vi "00 Main Simulated Signal (x64-2018).vi"() -> ()   [LabVIEW 2017]
panel:
  out "Error out (DAQ Loop)":errorcluster
  out "DAQ Loop Iterations":i32
  out "Raw DAQ Output":dynamicdata(graph)=[{"t0"=timestamp(3367839419.335167 s since 1904-01-01), "dt"=0.00016666666666666663, "Y"=array[240 elements], "attributes"=variant("NI_ChannelName"=variant(string "Voltage_0"), "NI_UnitDescription"=variant(string "Volts"))}, {"t0"=timestamp(3367839419.3351874 s since 1904-01-01), "dt"=0.00016666666666666663, "Y"=array[240 elements], "attributes"=variant("NI_ChannelName"=variant(string "Voltage_1"), "NI_UnitDescription"=variant(string "Volts"))}, {"t0"=timestamp(3367839419.3352084 s since 1904-01-01), "dt"=0.00016666666666666663, "Y"=array[240 elements], "attributes"=variant("NI_ChannelName"=variant(string "Voltage_2"), "NI_UnitDescription"=variant(string "Volts"))}]
  in  "All Stop!":bool
  out "Frequency 2":dynamicdata(graph)=[{"t0"=timestamp(3424329819.6880417 s since 1904-01-01), "dt"=0.00016666666666666663, "Y"=[50.00644377121546], "attributes"=variant("NI_ChannelName"=variant(string "Detected Frequency"))}, {"t0"=timestamp(3424329819.6880627 s since 1904-01-01), "dt"=0.00016666666666666663, "Y"=[49.993846178541475], "attributes"=variant("NI_ChannelName"=variant(string "Detected Frequency"))}, {"t0"=timestamp(3424329819.6880836 s since 1904-01-01), "dt"=0.00016666666666666663, "Y"=[49.994041382621866], "attributes"=variant("NI_ChannelName"=variant(string "Detected Frequency"))}] caption="Frequency"
  out "Phase 2":dynamicdata(graph)=[{"t0"=timestamp(3424329819.6880417 s since 1904-01-01), "dt"=0.00016666666666666663, "Y"=[-19.090260250465658], "attributes"=variant("NI_ChannelName"=variant(string "Detected Phase"))}, {"t0"=timestamp(3424329819.6880627 s since 1904-01-01), "dt"=0.00016666666666666663, "Y"=[-138.45601955575555], "attributes"=variant("NI_ChannelName"=variant(string "Detected Phase"))}, {"t0"=timestamp(3424329819.6880836 s since 1904-01-01), "dt"=0.00016666666666666663, "Y"=[102.37498697247455], "attributes"=variant("NI_ChannelName"=variant(string "Detected Phase"))}] caption="Frequency"
  out "Frequency":dbl format="%.2f"
  out "Amplitude":dbl format="%.2f"
  out "Phase":dbl format="%.2f"
  out "Acquisition Time":timestamp
  out "Voltage Waveform":dynamicdata(graph)=[{"t0"=timestamp(3424329819.638042 s since 1904-01-01), "dt"=0.00016666666666666663, "Y"=array[300 elements]}, {"t0"=timestamp(3424329819.6380625 s since 1904-01-01), "dt"=0.00016666666666666663, "Y"=array[300 elements]}, {"t0"=timestamp(3424329819.6380835 s since 1904-01-01), "dt"=0.00016666666666666663, "Y"=array[300 elements]}]
  out "IP":string
  out "Port":i32
  out "Transmitted Data":string
  out "Stop":bool
  out "Elements in Acquisition Buffer":i32
  # "V1.2 - PFI0 (Three Phase)"
  # "50.5"
  # "Rate"
  # "49.5"
  # "The code and design of this VI are licensed \nunder the terms of the New BSD License.\nPlease see the VI documentation or License.txt\nfor more details.\n\nCopyright (c) 2012, David Laverty\nwww.OpenPMU.org"
  # "180"
  # "-180"
  # "Configuration Information:\n\nThe ID and IP address to which the OpenPMU sends data is configured by 'C:\\PMUconfig.ini'.  If this doesn't exist, create it.\n\nCopy and paste the blue text below without the dashed lines into PMUconfig.ini.\n\n[Telecoms]\nID=PMU123\nIP=192.168.1.100\nPort=40001\n\nIP and Port may be any values within normal IPv4 range.  ID should be six alpha-numeric characters."
  # "Debug Stuff ( you're not supposed to find this :P )"
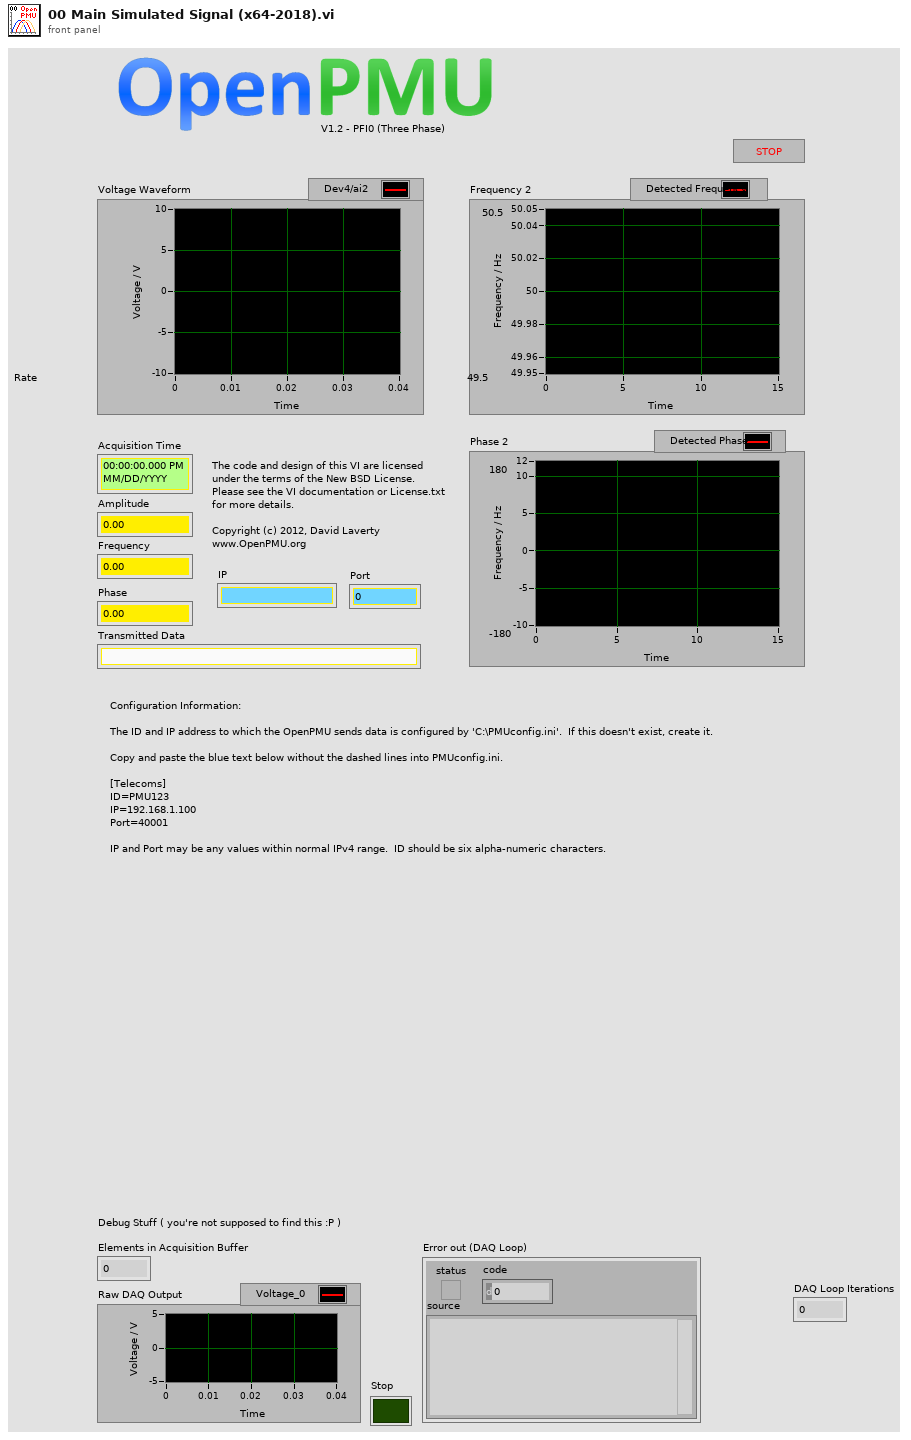
[diagram p1: front panel]
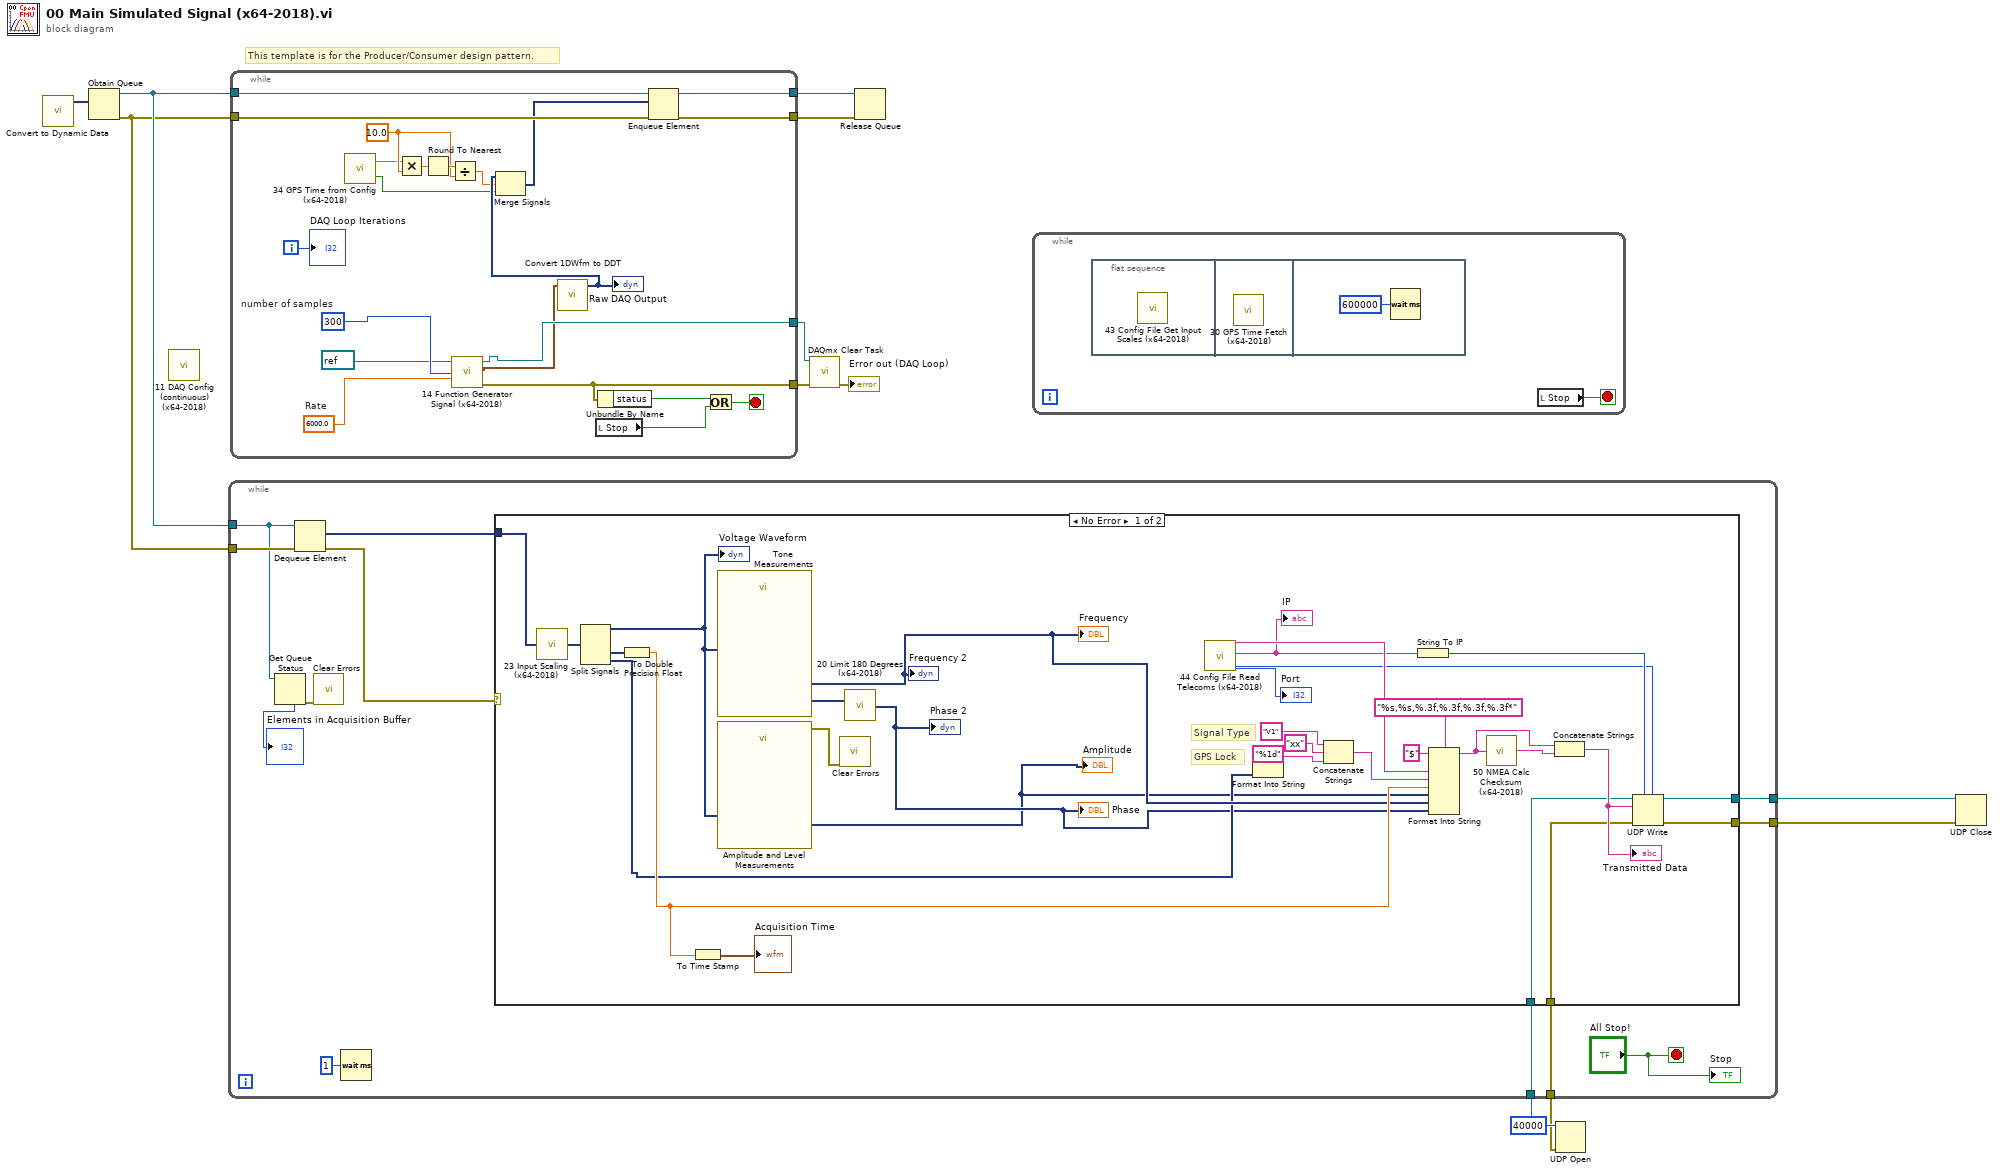
[diagram p0: block diagram]
diagram:
  # "This template is for the Producer/Consumer design pattern."
  n1 = call "Convert to Dynamic Data"() -> ("Dynamic Data Type"=w10:dynamicdata)  [unwired: 4 in]
  n2 = Obtain Queue(element data type=w10) -> (queue out=w7:refnum<queue>, error out=w6:errorcluster)  [unwired: 4 in, 1 out]
  n3 = call "11 DAQ Config (continuous) (x64-2018).vi"() -> ()  [unwired: 1 in, 2 out]
  n4 = while {
    tunnel: [w19] -> w13
    tunnel: [w17] -> w12
    tunnel: w7 -> [w31]
    tunnel: w6 -> [w30]
    tunnel: [w29] -> w9
    tunnel: [w28] -> w8
    i -> [w34]
    stop <- w33 stop-if-true
    w22 = 10.0 ("y")
    w16 = 6000.0  # Rate
    w15 = 300  # number of samples
    n5 = call "34 GPS Time from Config (x64-2018).vi"() -> ("GPS Lock"=w20:bool, "Time"=w21:dbl)  [unwired: 2 in]
    n6 = Multiply(x=w21, y=w22) -> (x*y=w25:dbl)
    n7 = Round To Nearest(number=w25) -> (nearest integer value=w24:dbl)
    n8 = Divide(x=w24, y=w22) -> (x/y=w23:dbl)
    n9 = call "14 Function Generator Signal (x64-2018).vi"("Rate"=w16, "Number of samples per channel"=w15, "task/channels in"=refnum<k21> refnum ("DAQmx Task Name")) -> ("Error Out"=w17:errorcluster, "data"=w18:waveform(dbl)[], "task out"=w19:refnum<k21>)  [unwired: 6 in]
    n10 = call <vilib>:"Convert 1DWfm to DDT.vi"("Array of Waveforms"=w18) -> ("Dynamic Data Type"=w27:dynamicdata)  [unwired: 3 in]
    "Raw DAQ Output" <- w27
    n11 = Merge Signals(w27, w23, w20) -> (w26:dynamicdata)
    n12 = local read "Stop"() -> (w32:bool)
    n13 = Unbundle By Name(w17) -> ("status"=w35:bool)
    n14 = Enqueue Element(queue=w31, element=w26, error in (no error)=w30) -> (queue out=w29:refnum<queue>, error out=w28:errorcluster)  [unwired: 1 in, 1 out]
    n15 = Or(x=w35, y=w32) -> (x .or. y?=w33:bool)
    "DAQ Loop Iterations" <- w34
  }
  n16 = call <vilib>:"DAQmx Clear Task.vi"("task in"=w13, "error in"=w12) -> ("error out"=→"Error out (DAQ Loop)":errorcluster)  [unwired: 13 in]
  n17 = Release Queue(queue=w9, error in (no error)=w8) -> ()  [unwired: 1 in, 3 out]
  n18 = while {
    stop <- w36 stop-if-true
    n19 = flat-sequence {
      frame #0 {
        n20 = call "43 Config File Get Input Scales (x64-2018).vi"() -> ()  [unwired: 1 in]
      }
      frame #1 {
        n21 = call "30 GPS Time Fetch (x64-2018).vi"() -> ()  [unwired: 1 in]
      }
      frame #2 {
        n22 = Wait (ms)(milliseconds to wait=u32 600000) -> ()  [unwired: 1 out]
      }
    }
    n23 = local read "Stop"() -> (w36:bool)
  }
  n24 = UDP Open(11:u16 40000 ("port")) -> (port=w4:refnum<k16>, 0:w3:errorcluster)  [unwired: 4 in, 1 out]
  n25 = while {
    tunnel: w7 -> [w43]
    tunnel: w6 -> [w45]
    tunnel: w4 -> [w42]
    tunnel: w3 -> [w41]
    tunnel: [w40] -> w2
    tunnel: [w39] -> w1
    stop <- "All Stop!" stop-if-true
    n26 = Get Queue Status(queue=w43) -> (error out=w38:errorcluster, # elements in queue=→"Elements in Acquisition Buffer":i32)  [unwired: 2 in, 6 out]
    n27 = Dequeue Element(queue=w43, error in (no error)=w45) -> (element=w46:dynamicdata, error out=w47:errorcluster)  [unwired: 1 in, 2 out]
    n28 = call <vilib>:"Clear Errors.vi"("error in (no error)"=w38) -> ()  [unwired: 5 in, 2 out]
    n29 = Wait (ms)(milliseconds to wait=u32 1) -> ()  [unwired: 1 out]
    n30 = case shown="No Error" w47 {
      tunnel: w46 -> [w56 _]
      tunnel: w42 -> [w73 w81]
      tunnel: w41 -> [w72 w80]
      tunnel: [w71 w81] -> w40
      tunnel: [w70 w80] -> w39
      frame No Error {
        # "GPS Lock"
        # "Signal Type"
        n31 = call "23 Input Scaling (x64-2018).vi"("Input (Raw)"=w56) -> ("Output (Scaled)"=w55:dynamicdata)
        n32 = Split Signals(w55) -> (w54:dynamicdata, w69:dynamicdata, w52:dynamicdata)  [unwired: 5 in, 2 out]
        "Voltage Waveform" <- w54
        n33 = To Double Precision Float(number=w69) -> (double precision float=w68:dbl)
        n34 = To Time Stamp(1:w68) -> (0:→"Acquisition Time":timestamp)
        n35 = call "Tone Measurements"("Signals"=w54) -> ("Phase"=w62:dynamicdata, "Frequency"=w53:dynamicdata)  [unwired: 7 in, 2 out]
        "Frequency 2" <- w53
        "Frequency" <- w53
        n36 = call "Amplitude and Level Measurements"("Signals"=w54) -> ("Cycle RMS"=w50:dynamicdata, "error out"=w79:errorcluster)  [unwired: 13 in]
        "Amplitude" <- w50
        n37 = call <vilib>:"Clear Errors.vi"("error in (no error)"=w79) -> ()  [unwired: 5 in, 2 out]
        n38 = call "20 Limit 180 Degrees (x64-2018).vi"("Angle In"=w62) -> ("Angle Out"=w51:dynamicdata)
        "Phase 2" <- w51
        "Phase" <- w51
        n39 = call "44 Config File Read Telecoms (x64-2018).vi"() -> ("Port"=w57:i32, "IP"=w58:string, "ID"=w59:string)  [unwired: 3 in]
        "IP" <- w58
        "Port" <- w57
        n40 = Format Into String(format string="%1d", w52) -> (resulting string=w63:string)  [unwired: 2 in, 1 out]
        n41 = Concatenate Strings("V1" ("input 2"), "xx" ("string"), w63) -> (w65:string)
        n42 = String To IP(1:w58) -> (0:w75:u32)
        n43 = Format Into String(format string="%s,%s,%.3f,%.3f,%.3f,%.3f*", initial string="$", w59, w65, w68, w50, w53, w51) -> (resulting string=w61:string)  [unwired: 1 in, 1 out]
        n44 = call "50 NMEA Calc Checksum (x64-2018).vi"("GPS String"=w61) -> ("hex integer string"=w60:string)  [unwired: 1 in, 1 out]
        n45 = Concatenate Strings(w61, w60) -> (w74:string)
        "Transmitted Data" <- w74
        n46 = UDP Write(address=w75, port or service name=w57, connection ID=w73, data in=w74, 8:w72) -> (error out=w70:errorcluster, 3:w71:refnum<k16>)  [unwired: 1 in]
      }
      frame Error {
      }
    }
    "Stop" <- "All Stop!"
  }
  n47 = UDP Close(connection ID=w2, 8:w1) -> ()  [unwired: 2 out]
